vi "OP500Z8P_ReadFromPDU.vi"(8 "errin":errorcluster, 10 "SN":string, 11 "VISA ITECH Name ?":refnum<visa-resource-name>) -> (0 "errout":errorcluster, 2 "All Data":string[](array[string]), 3 "BMS OK ?":bool)   [LabVIEW 2020]
uses:
  ZEN8 Semi Auto/OP500/VG/VG_progressBar.vi
  <vilib>/Utility/file.llb/Write Delimited Spreadsheet (string).vi
  <instrlib>/IT6000C/IT6000C.lvlib
  <userlib>/PCAN Basic/PCANBasic.lvlib
  <userlib>/PCAN Basic/Controls/BaudrateEenum.ctl
  <userlib>/PCAN Basic/Controls/Channel.ctl
  C:/Users/elhajj/OneDrive - FORSEE POWER/Bureau/Support banc de test/Ligne ZENPLUS/Code LabVIEW/CODE/02 SLIM ZEN WS 500/SubVi/FGV.ctl
  VG/VG_DCIR+OUIouNON_P.vi
  VG/VG_progressBar_P.vi
  VG/VG_DCIRCurrent_P.vi
panel:
  out "Stop":bool
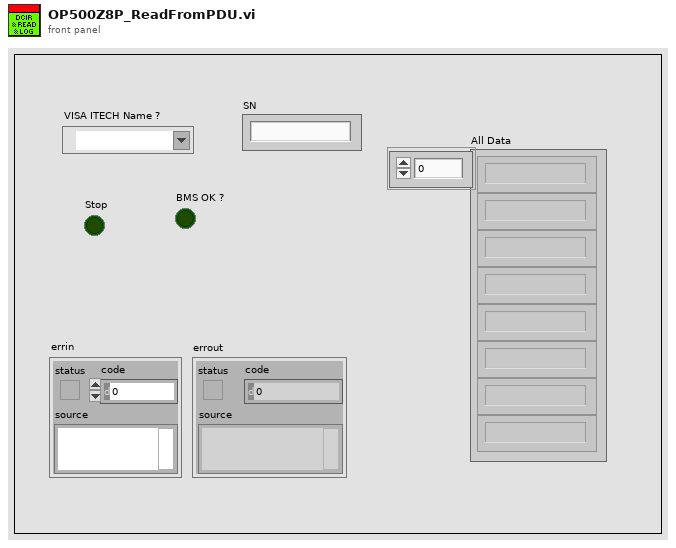
[diagram p1: front panel]
types:
  T1 = typedef "PCANBasic.lvlib/Channel.ctl" = enum16{"PCAN_NONEBUS", "not used1", "not used2", "not used3", "not used4", "not used5", "not used6", "not used7", "not used8", "not used9", "not used10", "not used11", "not used12", "not used13", "not used14", "not used15", "not used16", "not used17", "not used18", "not used19", "not used20", "not used21", "not used22", "not used23", "not used24", "not used25", "not used26", "not used27", "not used28", "not used29", "not used30", "not used31", "not used32", "PCAN_ISABUS1", "PCAN_ISABUS2", "PCAN_ISABUS3", "PCAN_ISABUS4", "PCAN_ISABUS5", "PCAN_ISABUS6", "PCAN_ISABUS7", "PCAN_ISABUS8", "not used41", "not used42", "not used43", "not used44", "not used45", "not used46", "not used47", "not used48", "PCAN_DNGBUS1", "not used50", "not used51", "not used52", "not used53", "not used54", "not used55", "not used56", "not used57", "not used58", "not used59", "not used60", "not used61", "not used62", "not used63", "not used64", "PCAN_PCIBUS1", "PCAN_PCIBUS2", "PCAN_PCIBUS3", "PCAN_PCIBUS4", "PCAN_PCIBUS5", "PCAN_PCIBUS6", "PCAN_PCIBUS7", "PCAN_PCIBUS8", "not used73", "not used74", "not used75", "not used76", "not used77", "not used78", "not used79", "not used80", "PCAN_USBBUS1", "PCAN_USBBUS2", "PCAN_USBBUS3", "PCAN_USBBUS4", "PCAN_USBBUS5", "PCAN_USBBUS6", "PCAN_USBBUS7", "PCAN_USBBUS8", "Not used89", "Not used90", "Not used91", "Not used92", "Not used93", "Not used94", "Not used95", "Not used96", "PCAN_PCCBUS1", "PCAN_PCCBUS2"}
  T2 = typedef "PCANBasic.lvlib/BaudrateEenum.ctl" = enum16{"CAN_Baud_1M", "CAN_Baud_800K", "CAN_BAUD_500K", "CAN_BAUD_250K", "CAN_BAUD_125K", "CAN_BAUD_100K", "CAN_BAUD_95K", "CAN_BAUD_83K", "CAN_BAUD_50K", "CAN_BAUD_47K", "CAN_BAUD_33K", "CAN_BAUD_20K", "CAN_BAUD_10K", "CAN_BAUD_5K", "User Baudrate"}
  T3 = typedef "FGV.ctl" = enum16{"GET", "SET", "RAZ"}
  T4 = typedef "PCANBasic.lvlib/CAN MSG Cluster.ctl" = cluster{"ID":u32, "MSG type":enum8{"STD", "RTR", "XTD", "XTD RTR", "STATUS"}, "LEN":i8, "DATA":u8[]}
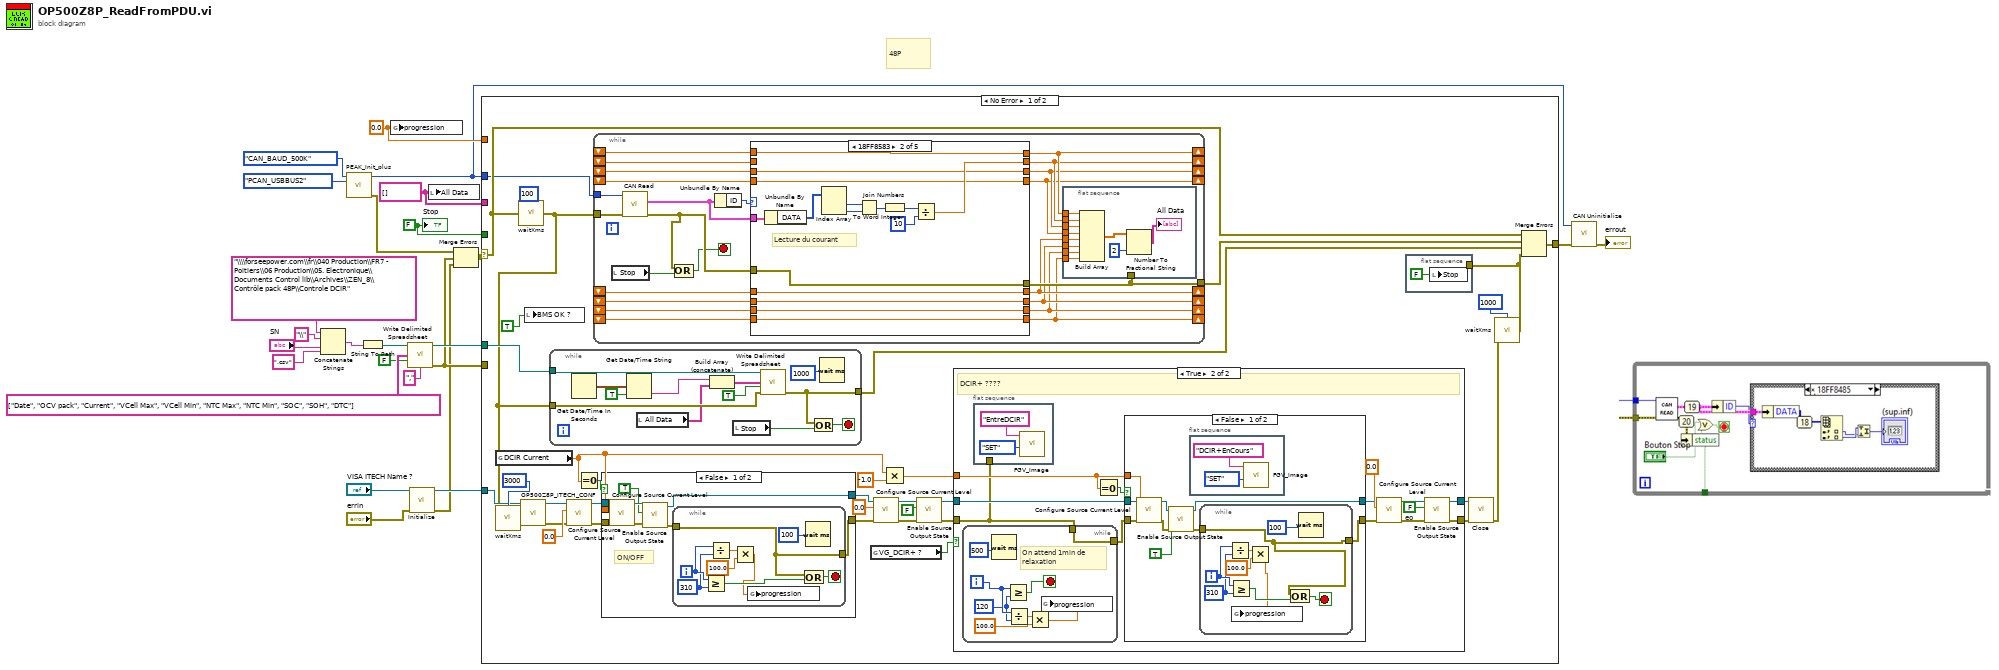
[diagram p0: block diagram]
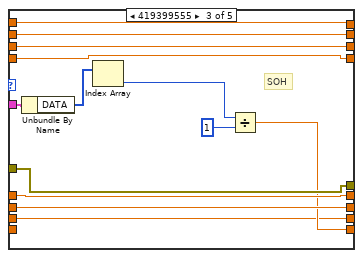
[diagram p3: hidden frame]
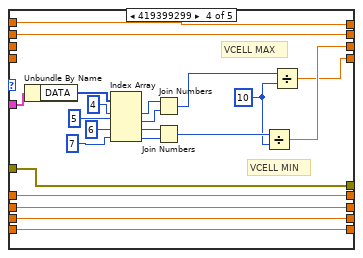
[diagram p4: hidden frame]
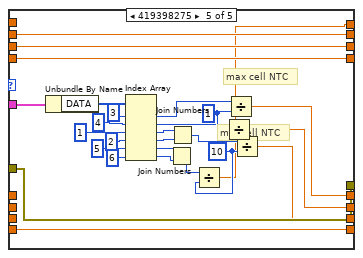
[diagram p5: hidden frame]
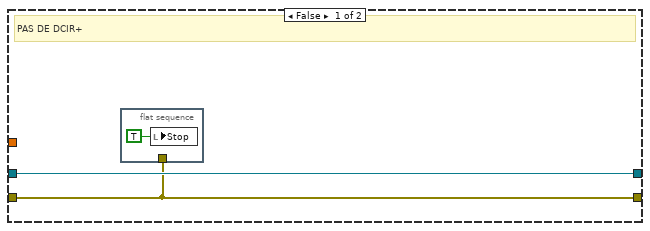
[diagram p7: hidden frame]
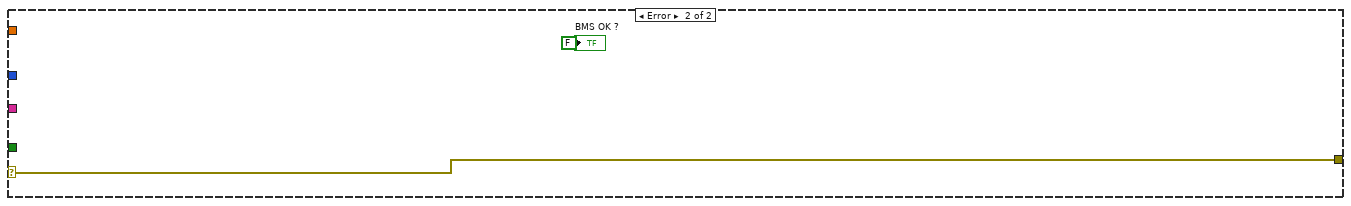
[diagram p9: hidden frame]
diagram:
  w8 = FALSE ("Stop")
  w19 = 0.0 ("progression")
  w20 = string[] []
  # "48P"
  n1 = Concatenate Strings("\\\\forseepower.com\\fr\\040 Production\\FR7 - Poitiers\\06 Production\\05. Electronique\\Documents Control lib\\Archives\\ZEN_8\\Contrôle pack 48P\\Controle DCIR" ("chaîne"), "\\" ("chaîne"), "SN", ".csv" ("chaîne")) -> (w10:string)
  n2 = call <userlib>:"PEAK_Init_plus.vi"("Channel"=Channel."PCAN_USBBUS2", "BTR0BTR1"=BaudrateEenum."CAN_BAUD_500K") -> ("errout"=w1:errorcluster, "Channel out"=w2:T1)  [unwired: 8 in]
  n3 = String To Path(string=w10) -> (path=w11:path)
  n4 = global write "VG_progressBar.vi" "progression"(w19) -> ()
  n5 = call-poly <vilib>:"Write Delimited Spreadsheet.vi"("file path (dialog if empty)"=w11, "1D data"=string[] ["Date", "OCV pack", "Current", "VCell Max", "VCell Min", "NTC Max", "NTC Min", "SOC", "SOH", "DTC"], "append to file? (new file:F)"=FALSE, "delimiter (\\t)"="," ("delimiter (\\t)")) -> ("new file path (Not A Path if cancelled)"=w24:path, "error out"=w21:errorcluster)  [unwired: 10 in]
  n6 = call <instrlib>:"Initialize.vi"("error in (no error)"="errin", "VISA resource name"="VISA ITECH Name ?") -> ("error out"=w16:errorcluster, "VISA resource name out"=w17:refnum<visa-resource-name>)  [unwired: 8 in]
  n7 = local write "All Data"(w20) -> ()
  n8 = Merge Errors(w1, w21, w16) -> (w22:errorcluster)
  n9 = case shown="No Error" w22 {
    selector: w22 -> [w54 w265]
    tunnel: [w60 w265] -> w6
    tunnel: w24 -> [w55 _]
    tunnel: w21 -> [_ _]
    tunnel: w20 -> [_ _]
    tunnel: w19 -> [_ _]
    tunnel: w17 -> [w39 _]
    tunnel: w8 -> [_ _]
    tunnel: w2 -> [w30 _]
    frame No Error {
      n10 = global read "VG_DCIRCurrent_P.vi" "DCIR Current"() -> (w26:dbl)
      n11 = call <userlib>:"waitXms.vi"("attente (ms)"=u32 100, "errin"=w54) -> ("errout"=w32:errorcluster)  [unwired: 13 in]
      n12 = call <userlib>:"waitXms.vi"("attente (ms)"=u32 3000, "errin"=w32) -> ("errout"=w41:errorcluster)  [unwired: 13 in]
      n13 = call "OP500Z8P_ITECH_CONF.vi"("ErrIN"=w41, "VISAin"=w39) -> ("ErrOUT"=w40:errorcluster, "VisaOUT"=w38:refnum<visa-resource-name>)  [unwired: 8 in]
      n14 = local write "BMS OK ?"(TRUE ("BMS OK ?")) -> ()
      n15 = while {
        tunnel: w55 -> [w258]
        tunnel: w32 -> [w257]
        tunnel: [w252] -> w49
        stop <- w254 stop-if-true
        n16 = Get Date/Time In Seconds() -> (seconds since 1Jan1904=w262:timestamp)
        n17 = Get Date/Time String(seconds (now)=w262, want seconds? (F)=TRUE ("secondes ? (F)")) -> (time string=w256:string)  [unwired: 1 in, 1 out]
        n18 = local read "All Data"() -> (w255:string[])
        n19 = Build Array (concatenate)(w256, w255) -> (w260:string[])
        n20 = local read "Stop"() -> (w253:bool)
        n21 = call-poly <vilib>:"Write Delimited Spreadsheet.vi"("file path (dialog if empty)"=w258, "1D data"=w260, "append to file? (new file:F)"=TRUE, "error in (no error)"=w257) -> ("error out"=w252:errorcluster)  [unwired: 10 in, 1 out]
        n22 = Compound Arithmetic op=OR ("Opérateur arithmétique")(w252, w253) -> (w254:bool)
        n23 = Wait (ms)(milliseconds to wait=u32 1000 ("attente (ms)")) -> ()  [unwired: 1 out]
      }
      n24 = call <instrlib>:"Configure Source Current Level.vi"("error in (no error)"=w40, "Value(0)"=0.0, "VISA resource name"=w38) -> ("error out"=w36:errorcluster, "VISA resource name out"=w37:refnum<visa-resource-name>)  [unwired: 7 in]
      n25 = Equal To 0?(x=w26) -> (x = 0?=w35:bool)
      n26 = while {
        tunnel: w32 -> [w85]
        tunnel: [w82] -> w31
        tunnel: w30 -> [w79]
        shift-right: [w78] -> _
        shift-left: _ -> [w77]
        shift-right: [w76] -> _
        shift-left: _ -> [w75]
        shift-right: [w74] -> _
        shift-left: _ -> [w73]
        shift-right: [w63] -> _
        shift-left: _ -> [w72]
        shift-right: [w69] -> _
        shift-left: _ -> [w71]
        shift-right: [w68] -> _
        shift-left: _ -> [w70]
        shift-right: [w67] -> _
        shift-left: _ -> [w65]
        shift-right: [w66] -> _
        shift-left: _ -> [w64]
        stop <- w80 stop-if-true
        n27 = local read "Stop"() -> (w62:bool)
        n28 = call <userlib>:"CAN Read.vi"("error in (no error)"=w85, "Channel"=w79) -> ("error out"=w81:errorcluster, "CAN_Message out"=w83:T4)  [unwired: 5 in, 3 out]
        n29 = Compound Arithmetic op=OR ("Opérateur arithmétique")(w81, w62) -> (w80:bool)
        n30 = Unbundle By Name(w83) -> ("ID"=w84:u32)
        n31 = case shown="18FF8583" w84 {
          tunnel: w83 -> [_ w121 w134 w156 w183]
          tunnel: w81 -> [w105 w116 w132 w151 w181]
          tunnel: [w105 w116 w132 w151 w181] -> w82
          tunnel: [w104 w114 w123 w150 w157] -> w78
          tunnel: [w103 w115 w130 w149 w180] -> w76
          tunnel: [w102 w113 w129 w138 w179] -> w74
          tunnel: w77 -> [w104 w114 w123 w150 _]
          tunnel: w75 -> [w103 _ w130 w149 w180]
          tunnel: w73 -> [w102 w113 w129 _ w179]
          tunnel: [w101 w112 w128 w137 w178] -> w63
          tunnel: w72 -> [w101 w112 w128 _ w178]
          tunnel: [w100 w111 w127 w148 w172] -> w69
          tunnel: [w99 w110 w126 w147 w171] -> w68
          tunnel: w71 -> [w100 w111 w127 w148 _]
          tunnel: w70 -> [w99 w110 w126 w147 _]
          tunnel: [w98 w109 w124 w146 w164] -> w67
          tunnel: [w97 w108 w125 w145 w170] -> w66
          tunnel: w65 -> [w98 w109 w124 w146 _]
          tunnel: w64 -> [w97 w108 _ w145 w170]
          frame 0, Default {
          }
          frame 419399043 {
            # "Lecture du courant"
            n32 = Unbundle By Name(w121) -> ("DATA"=w120:u8[])
            n33 = Index Array(array=w120) -> (element #1=w107:u8, element #2=w106:u8)  [unwired: 2 in]
            n34 = Join Numbers(hi=w107, lo=w106) -> ((hi.lo)=w118:u16)
            n35 = To Word Integer(number=w118) -> (16bit integer=w117:i16)
            n36 = Divide(x=w117, y=u16 10) -> (x/y=w115:dbl)
          }
          frame 419399555 {
            # "SOH"
            n37 = Unbundle By Name(w134) -> ("DATA"=w133:u8[])
            n38 = Index Array(array=w133) -> (element=w122:u8)  [unwired: 1 in]
            n39 = Divide(x=w122, y=u8 1) -> (x/y=w125:dbl)
          }
          frame 419399299 {
            w152 = u16 10 ("y")
            # "VCELL MIN"
            # "VCELL MAX"
            n40 = Unbundle By Name(w156) -> ("DATA"=w155:u8[])
            n41 = Index Array(array=w155, index #1=4 ("index"), index #2=5 ("index"), index #3=6 ("index"), index #4=7 ("index")) -> (element #1=w142:u8, element #2=w141:u8, element #3=w136:u8, element #4=w135:u8)
            n42 = Join Numbers(hi=w142, lo=w141) -> ((hi.lo)=w154:u16)
            n43 = Join Numbers(hi=w136, lo=w135) -> ((hi.lo)=w153:u16)
            n44 = Divide(x=w153, y=w152) -> (x/y=w138:dbl)
            n45 = Divide(x=w154, y=w152) -> (x/y=w137:dbl)
          }
          frame 419398275 {
            w158 = u16 10 ("y")
            w174 = u8 1 ("y")
            # "min cell NTC"
            # "max cell NTC"
            n46 = Unbundle By Name(w183) -> ("DATA"=w182:u8[])
            n47 = Index Array(array=w182, index #1=3 ("index"), index #2=4 ("index"), index #3=1 ("index"), index #4=2 ("index"), index #5=5 ("index"), index #6=6 ("index")) -> (element #1=w177:u8, element #2=w173:u8, element #3=w167:u8, element #4=w166:u8, element #5=w161:u8, element #6=w160:u8)
            n48 = Join Numbers(hi=w161, lo=w160) -> ((hi.lo)=w159:u16)
            n49 = Join Numbers(hi=w167, lo=w166) -> ((hi.lo)=w165:u16)
            n50 = Divide(x=w159, y=w158) -> (x/y=w157:dbl)
            n51 = Divide(x=w173, y=w174) -> (x/y=w171:dbl)
            n52 = Divide(x=w177, y=w174) -> (x/y=w172:dbl)
            n53 = Divide(x=w165, y=w158) -> (x/y=w164:dbl)
          }
        }
        n54 = flat-sequence {
          tunnel: w82 -> [_]
          tunnel: w78 -> [w94]
          tunnel: w76 -> [w93]
          tunnel: w74 -> [w92]
          tunnel: w69 -> [w91]
          tunnel: w68 -> [w90]
          tunnel: w67 -> [w89]
          tunnel: w66 -> [w88]
          tunnel: w63 -> [w87]
          frame #0 {
            n55 = Build Array(w94, w93, w92, w87, w91, w90, w89, w88) -> (w95:dbl[])
            n56 = Number To Fractional String(number=w95, precision (6)=i16 2 ("précision (6)")) -> (F-format string=→"All Data":string[])  [unwired: 2 in]
          }
        }
      }
      n57 = case shown="False" w35 {
        tunnel: w37 -> [w188 w203]
        tunnel: w36 -> [w187 w202]
        tunnel: w26 -> [w186 _]
        tunnel: [w185 w203] -> w34
        tunnel: [w184 w202] -> w33
        frame False {
          # "ON/OFF"
          n58 = call <instrlib>:"Configure Source Current Level.vi"("error in (no error)"=w187, "Value(0)"=w186, "VISA resource name"=w188) -> ("error out"=w192:errorcluster, "VISA resource name out"=w191:refnum<visa-resource-name>)  [unwired: 7 in]
          n59 = call <instrlib>:"Enable Source Output State.vi"("error in (no error)"=w192, "Enable(True)"=TRUE, "VISA resource name"=w191) -> ("error out"=w189:errorcluster, "VISA resource name out"=w185:refnum<visa-resource-name>)  [unwired: 7 in]
          n60 = while {
            tunnel: w189 -> [w194]
            tunnel: [w194] -> w184
            i -> [w199]
            stop <- w195 stop-if-true
            w198 = 310 ("y")
            n61 = Greater Or Equal?(x=w199, y=w198) -> (x >= y?=w200:bool)
            n62 = Divide(x=w199, y=w198) -> (x/y=w197:dbl)
            n63 = Multiply(x=w197, y=100.0) -> (x*y=w193:dbl)
            n64 = global write "VG_progressBar_P.vi" "progression"(w193) -> ()
            n65 = Compound Arithmetic op=OR ("Opérateur arithmétique")(w194, w200) -> (w195:bool)
            n66 = Wait (ms)(milliseconds to wait=u32 100 ("attente (ms)")) -> ()  [unwired: 1 out]
          }
        }
        frame True {
        }
      }
      n67 = global read "VG_DCIR+OUIouNON_P.vi" "VG_DCIR+ ?"() -> (w42:bool)
      n68 = call <instrlib>:"Configure Source Current Level.vi"("error in (no error)"=w33, "Value(0)"=0.0, "VISA resource name"=w34) -> ("error out"=w46:errorcluster, "VISA resource name out"=w45:refnum<visa-resource-name>)  [unwired: 7 in]
      n69 = Multiply(x=w26, y=-1.0) -> (x*y=w51:dbl)
      n70 = call <instrlib>:"Enable Source Output State.vi"("error in (no error)"=w46, "Enable(True)"=FALSE, "VISA resource name"=w45) -> ("error out"=w44:errorcluster, "VISA resource name out"=w43:refnum<visa-resource-name>)  [unwired: 7 in]
      n71 = case shown="True" w42 {
        tunnel: [w204 w215] -> w58
        tunnel: [w205 w214] -> w57
        tunnel: w51 -> [_ w210]
        tunnel: w44 -> [w204 w208]
        tunnel: w43 -> [w205 w212]
        frame False {
          # "PAS DE DCIR+"
          n72 = flat-sequence {
            tunnel: w204 -> [_]
            frame #0 {
              n73 = local write "Stop"(TRUE ("Stop")) -> ()
            }
          }
        }
        frame True {
          w219 = FALSE  # eo
          # "DCIR+ ????"
          n74 = while {
            tunnel: w208 -> [w226]
            tunnel: [w226] -> w207
            i -> [w224]
            stop <- w225 stop-if-true
            w223 = u32 120 ("attente (ms)")
            # "On attend 1min de\nrelaxation"
            n75 = Wait (ms)(milliseconds to wait=u32 500 ("attente (ms)")) -> ()  [unwired: 1 out]
            n76 = Greater Or Equal?(x=w224, y=w223) -> (x >= y?=w225:bool)
            n77 = Divide(x=w224, y=w223) -> (x/y=w222:dbl)
            n78 = Multiply(x=w222, y=100.0) -> (x*y=w220:dbl)
            n79 = global write "VG_progressBar_P.vi" "progression"(w220) -> ()
          }
          n80 = flat-sequence {
            tunnel: w208 -> [_]
            frame #0 {
              n81 = call "FGV_Image.vi"("Énum"=FGV."SET", "IN"="EntreDCIR") -> ()  [unwired: 9 in, 1 out]
            }
          }
          n82 = Equal To 0?(x=w210) -> (x = 0?=w209:bool)
          n83 = case shown="False" w209 {
            tunnel: [w228 w249] -> w213
            tunnel: w210 -> [w234 _]
            tunnel: w212 -> [w235 w249]
            tunnel: [w232 w248] -> w211
            tunnel: w207 -> [w236 w248]
            frame False {
              n84 = call <instrlib>:"Configure Source Current Level.vi"("error in (no error)"=w236, "Value(0)"=w234, "VISA resource name"=w235) -> ("error out"=w231:errorcluster, "VISA resource name out"=w229:refnum<visa-resource-name>)  [unwired: 7 in]
              n85 = call <instrlib>:"Enable Source Output State.vi"("error in (no error)"=w231, "Enable(True)"=TRUE, "VISA resource name"=w229) -> ("error out"=w230:errorcluster, "VISA resource name out"=w228:refnum<visa-resource-name>)  [unwired: 7 in]
              n86 = flat-sequence {
                frame #0 {
                  n87 = call "FGV_Image.vi"("Énum"=FGV."SET", "IN"="DCIR+EnCours") -> ()  [unwired: 9 in, 1 out]
                }
              }
              n88 = while {
                tunnel: w230 -> [w240]
                tunnel: [w240] -> w232
                i -> [w243]
                stop <- w241 stop-if-true
                w242 = u32 310 ("attente (ms)")
                n89 = Divide(x=w243, y=w242) -> (x/y=w245:dbl)
                n90 = Greater Or Equal?(x=w243, y=w242) -> (x >= y?=w246:bool)
                n91 = Multiply(x=w245, y=100.0) -> (x*y=w239:dbl)
                n92 = global write "VG_progressBar_P.vi" "progression"(w239) -> ()
                n93 = Compound Arithmetic op=OR ("Opérateur arithmétique")(w240, w246) -> (w241:bool)
                n94 = Wait (ms)(milliseconds to wait=u32 100 ("attente (ms)")) -> ()  [unwired: 1 out]
              }
            }
            frame True {
            }
          }
          n95 = call <instrlib>:"Configure Source Current Level.vi"("error in (no error)"=w211, "Value(0)"=0.0, "VISA resource name"=w213) -> ("error out"=w218:errorcluster, "VISA resource name out"=w217:refnum<visa-resource-name>)  [unwired: 7 in]
          n96 = call <instrlib>:"Enable Source Output State.vi"("error in (no error)"=w218, "Enable(True)"=w219, "VISA resource name"=w217) -> ("error out"=w215:errorcluster, "VISA resource name out"=w214:refnum<visa-resource-name>)  [unwired: 7 in]
        }
      }
      n97 = flat-sequence {
        tunnel: w27 -> [_]
        frame #0 {
          n98 = local write "Stop"(FALSE ("Stop")) -> ()
        }
      }
      n99 = call <instrlib>:"Close.vi"("error in (no error)"=w58, "VISA resource name"=w57) -> ("error out"=w28:errorcluster)  [unwired: 9 in]
      n100 = call <userlib>:"waitXms.vi"("attente (ms)"=u32 1000, "errin"=w28) -> ("errout"=w27:errorcluster)  [unwired: 13 in]
      n101 = Merge Errors(w54, w31, w49, w27) -> (w60:errorcluster)
    }
    frame Error {
      "BMS OK ?" <- FALSE ("BMS OK ?")
    }
  }
  n102 = call <userlib>:"CAN Uninitialize.vi"("error in (no error)"=w6, "Channel"=w2) -> ("error out"=→"errout":errorcluster)  [unwired: 7 in, 2 out]
  "Stop" <- w8
